vi "Write Nr.vi"(8 "error in (no error)":errorcluster, 9 "DG Nr":i32, 10 "Nr":i32, 11 "BME_DG_Chnl in":refnum<class "BME_DG_Chnl.lvclass">) -> (0 "error out":errorcluster, 3 "BME_DG_Chnl out":refnum<class "BME_DG_Chnl.lvclass">)   [LabVIEW 2009, in "POLARIS BME DG.lvlib" / "BME_DG_Chnl.lvclass"]
uses:
  BME_DG_Chnl.lvclass
  BME_DG_Chnl.lvclass/BME_DG_Chnl.ctl
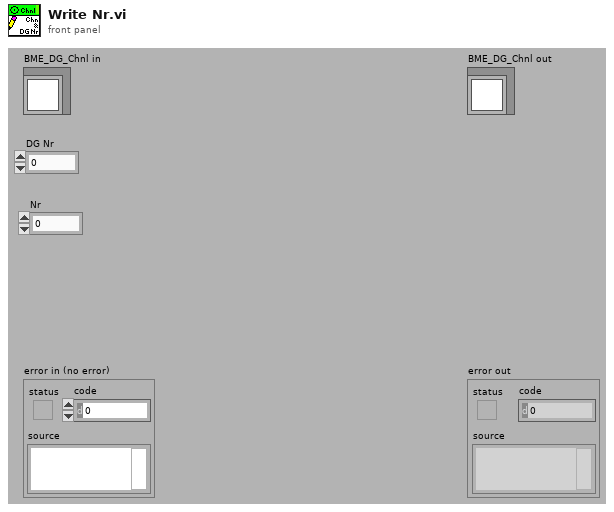
[diagram p1: front panel]
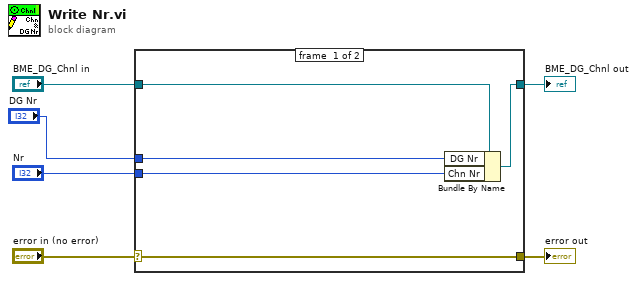
[diagram p0: block diagram]
diagram:
  n1 = case shown="No Error" "error in (no error)" {
    selector: "error in (no error)" -> [w11 w12]
    tunnel: [w11 w12] -> w5
    tunnel: [w9 w13] -> w3
    tunnel: "BME_DG_Chnl in" -> [w10 w13]
    tunnel: "Nr" -> [w8 _]
    tunnel: "DG Nr" -> [w7 _]
    frame #0 {
      n2 = Bundle By Name(cluster=w10, "DG Nr"=w7, "Chn Nr"=w8) -> (w9:refnum<class "BME_DG_Chnl.lvclass">)
    }
    frame #1 {
    }
  }
  "error out" <- w5
  "BME_DG_Chnl out" <- w3
